vi "Send Update Entity Details.vi"(5 "status":string, 7 "Message Priority (Normal)":T2=enum."Normal", 8 "error in (no error)":errorcluster, 9 "enqueuer":refnum<class "Message Enqueuer.lvclass">, 10 "Entity Type":T1, 11 "Message Enqueuer":refnum<class "Message Enqueuer.lvclass">) -> (0 "error out":errorcluster, 3 "Message Enqueuer out":refnum<class "Message Enqueuer.lvclass">)   [LabVIEW 2023, in "Coffee Shop.lvlib" / "Update Entity Details Msg.lvclass"]
doc: "This VI sends the message to an actor."
uses:
  Update Entity Details Msg.lvclass
  <vilib>/ActorFramework/Message Enqueuer/Message Enqueuer.lvclass
  <vilib>/ActorFramework/Message Enqueuer/Message Priority.ctl
  Coffee Shop/Entity Types.ctl
  c:/dev/_r/4/eng/lv-core/lvpostprocessingd/lv_mc_x86_64/dist_i386/vi.lib/ActorFramework/Message/Message.lvclass
  Update Entity Details Msg.lvclass/Update Entity Details Msg.ctl
  <vilib>/ActorFramework/Message Enqueuer/Message Enqueuer.lvclass/Message Enqueuer.ctl
  <vilib>/ActorFramework/Message Priority Queue/Priority Enqueue.vi
  Coffee Shop/Coffee Shop.lvclass
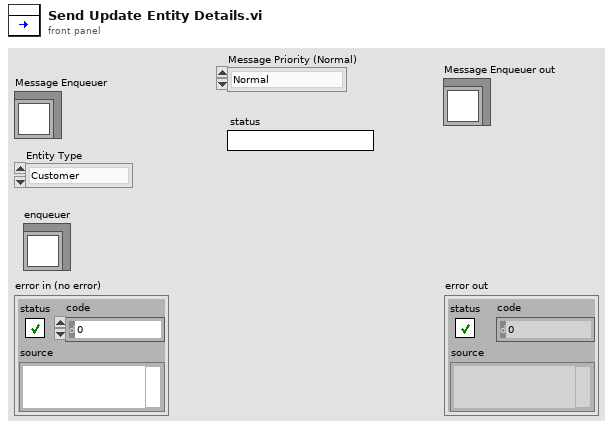
[diagram p1: front panel]
types:
  T1 = typedef "Coffee Shop.lvlib/Coffee Shop.lvclass/Entity Types.ctl" = enum16{"Customer", "Cashier", "Barista"}
  T2 = typedef "Actor Framework.lvlib/Message Enqueuer.lvclass/Message Priority.ctl" = enum16{"Low", "Normal", "High"}
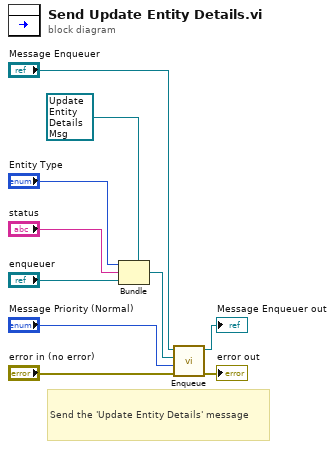
[diagram p0: block diagram]
diagram:
  # "Send the 'Update Entity Details' message"
  n1 = Bundle(cluster=refnum<class "Update Entity Details Msg.lvclass"> refnum ("Object"), "Entity Type", "status", "enqueuer") -> (w6:refnum<class "Update Entity Details Msg.lvclass">)
  n2 = call <vilib>:"Enqueue.vi"("error in (no error)"="error in (no error)", "Message Priority (Normal)"="Message Priority (Normal)", "Message"=w6, "Message Enqueuer in"="Message Enqueuer") -> ("error out"=→"error out":errorcluster, "Message Enqueuer out"=→"Message Enqueuer out":refnum<class "Message Enqueuer.lvclass">)  [unwired: 6 in]
